vi "GetEvtReports.vi"(8 "error in (no error)":errorcluster, 11 "C37EventPlugin in":refnum<class "C37Plugin.lvclass">) -> (0 "error out":errorcluster, 3 "C37EventPlugin out":refnum<class "C37Plugin.lvclass">)   [LabVIEW 2014, in "WfrmPlugins.lvlib" / "C37Plugin.lvclass"]
uses:
  C37Plugin.lvclass
  EventPluginBaseClass/TypeDefs/clEvtReport.ctl
  C:/Labview Data/MathScriptVIs/MCStatic_33564263232_cd0c74153415d248b874e5dd603eedc9.vi
  <instcachedir>/0/MCStatic_33564263232_cd0c74153415d248b874e5dd603eedc9_1BD6B912C34A4BF9A206F4FEB7E1A62C.lvgen/MCStatic_33564263232_cd0c74153415d248b874e5dd603eedc9_1BD6B912C34A4BF9A206F4FEB7E1A62C_000.vi
  <vilib>/imath/engines/lvmath2/RunTimeEngine/UserFunctionToken/NIMS_UserFunction_CondDefined.vi
  <instcachedir>/0/NIMS_UserFunction_CondDefined_359D6D699583402F98E5D4DB7FB40D41.lvgen/NIMS_UserFunction_CondDefined_359D6D699583402F98E5D4DB7FB40D41_000.vi
  <vilib>/imathl/engines/lvmath/Functions/Error Handling/Create Error.vi
  <vilib>/imath/engines/lvmath2/RunTimeEngine/VariableToken/NIMS_VariableToken_CondDefined.vi
  <instcachedir>/0/NIMS_VariableToken_CondDefined_EE8DD211A89249938CE6537267F5C9B3.lvgen/NIMS_VariableToken_CondDefined_EE8DD211A89249938CE6537267F5C9B3_004.vi
  <vilib>/imath/engines/lvmath/Functions/Error Handling/MergeErrorsWrapper.vi
  <vilib>/imath/engines/lvmath2/RunTimeEngine/NodeEndStatement/NIMS_NodeEndStatement_Output.vi
  <instcachedir>/0/NIMS_NodeEndStatement_Output_53EC0D466D134D7ABD903AC30B43404B.lvgen/NIMS_NodeEndStatement_Output_53EC0D466D134D7ABD903AC30B43404B_005.vi
  <instcachedir>/0/NIMS_NodeEndStatement_Output_53EC0D466D134D7ABD903AC30B43404B.lvgen/NIMS_NodeEndStatement_Output_53EC0D466D134D7ABD903AC30B43404B_003.vi
  <vilib>/imath/engines/lvmath2/RunTimeEngine/ErrorHandling/NIMS_Finalize Error.vi
  Matlab/C37/C37evt.m
  EventPluginBaseClass/BaseWfrmPlugin.lvclass
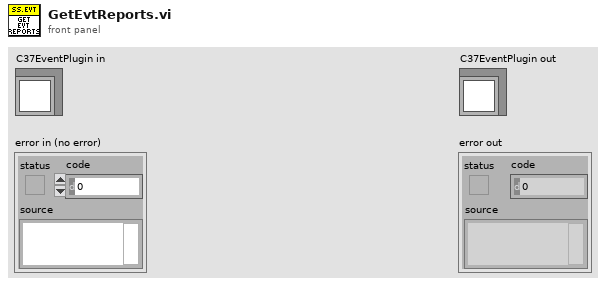
[diagram p1: front panel]
types:
  T1 = typedef "WfrmPlugins.lvlib/BaseWfrmPlugin.lvclass/clEvtReport.ctl" = cluster{"Timestamp":dbl, "Synx":cdb[], "Freq":dbl, "ROCOF":dbl}
  T2 = typedef "WfrmPlugins.lvlib/BaseWfrmPlugin.lvclass/WfrmConfig.ctl" = cluster{"T0(UTC)":dbl, "F0":dbl, "Fs":i32, "FSamp":u32}
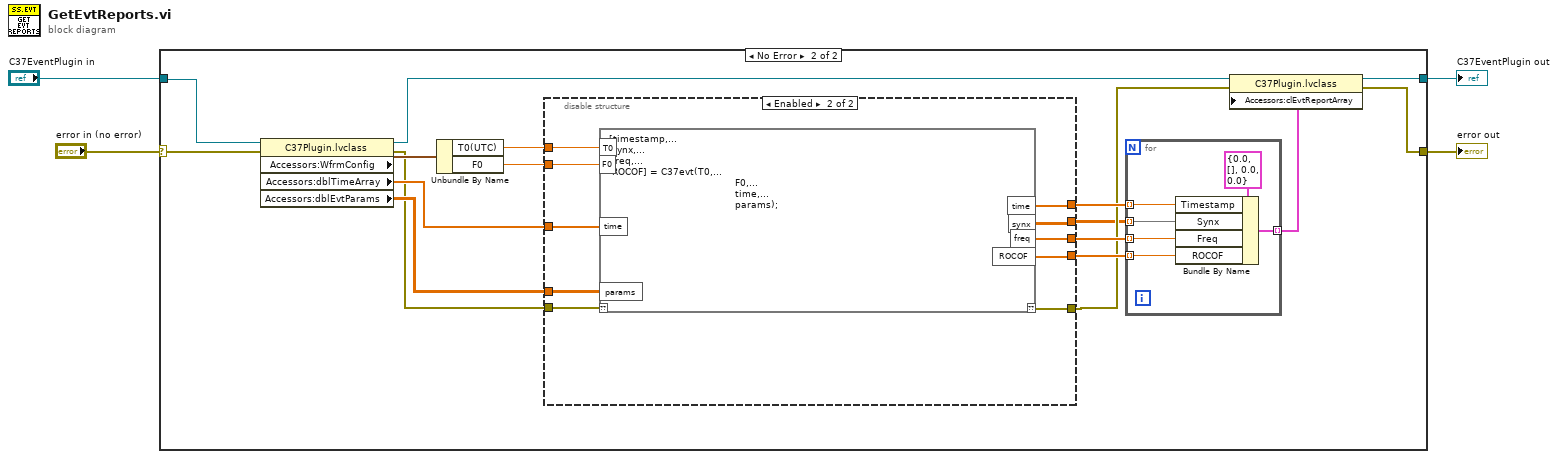
[diagram p0: block diagram]
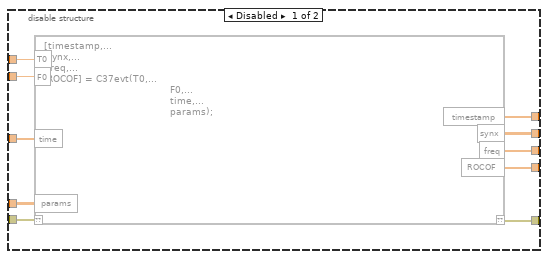
[diagram p3: hidden frame]
diagram:
  n1 = case shown="No Error" "error in (no error)" {
    selector: "error in (no error)" -> [w6 w18]
    tunnel: [w5 w21] -> w4
    tunnel: "C37EventPlugin in" -> [w5 w19]
    tunnel: [w6 w20] -> w3
    frame Error {
    }
    frame No Error {
      n2 = property class="C37Plugin.lvclass"(reference=w19, error in=w18) -> (reference out=w14:refnum<class "C37Plugin.lvclass">, error out=w7:errorcluster, "Accessors:WfrmConfig"=w17:T2, "Accessors:dblTimeArray"=w9:dbl[], "Accessors:dblEvtParams"=w8:dbl[][])
      n3 = Unbundle By Name(w17) -> ("T0(UTC)"=w16:dbl, "F0"=w15:dbl)
      n4 = disable-structure shown="Enabled" {
        disable-tunnel: [w33 w35] -> w23
        disable-tunnel: [w32 w34] -> w22
        disable-tunnel: w16 -> [w31 w43]
        disable-tunnel: w15 -> [w30 w42]
        disable-tunnel: [w29 w37] -> w13
        disable-tunnel: [w28 w38] -> w12
        disable-tunnel: [w27 w36] -> w11
        disable-tunnel: w9 -> [w26 w41]
        disable-tunnel: w8 -> [w25 w40]
        disable-tunnel: w7 -> [w24 w39]
        frame Disabled {
          n5 = script code="[timestamp,...\n synx,...\n freq,...\n ROCOF] = C37evt(T0,...\n                                          F0,...\n                                          time,...\n                                          params);"("??"=w24, "T0"=w31, "F0"=w30, "time"=w26, "params"=w25) -> ("??"=w28:errorcluster, "timestamp"=w29:dbl[], "synx"=w27:cdb[][], "freq"=w33:dbl[], "ROCOF"=w32:dbl[])
        }
        frame Enabled {
          n6 = mathscript code="[timestamp,...\n synx,...\n freq,...\n ROCOF] = C37evt(T0,...\n                                          F0,...\n                                          time,...\n                                          params);"("??"=w39, "T0"=w43, "F0"=w42, "time"=w41, "params"=w40) -> ("??"=w38:errorcluster, "synx"=w36:cdb[][], "time"=w37:dbl[], "freq"=w35:dbl[], "ROCOF"=w34:dbl[])
        }
      }
      n7 = for {
        tunnel: w13 -> [w133] mode=indexing
        tunnel: w23 -> [w132] mode=indexing
        tunnel: w22 -> [w131] mode=indexing
        tunnel: [w129] -> w10 mode=indexing
        tunnel: w11 -> [w128] mode=indexing
        n8 = Bundle By Name(cluster=T1 {"Timestamp"=0.0, "Synx"=[], "Freq"=0.0, "ROCOF"=0.0} ("clReport"), "Timestamp"=w133, "Synx"=w128, "Freq"=w132, "ROCOF"=w131) -> (w129:T1)
      }
      n9 = property class="C37Plugin.lvclass"(reference=w14, error in=w12, "Accessors:clEvtReportArray"=w10) -> (reference out=w21:refnum<class "C37Plugin.lvclass">, error out=w20:errorcluster)
    }
  }
  "error out" <- w3
  "C37EventPlugin out" <- w4
